vi "Write OCP_Enable.vi"(8 "error in":errorcluster, 10 "OCP_Enable":bool, 11 "36234A in":refnum<class "36234A.lvclass">) -> (0 "error out":errorcluster, 3 "36234A out":refnum<class "36234A.lvclass">)   [LabVIEW 2019, in "36234A.lvlib" / "36234A.lvclass"]
uses:
  Library/36234A.lvclass
  C:/Users/Public/Documents/Development/builds/Instruments/PowerSupply.lvlibp/Library/PowerSupply.lvclass
  Library/36234A.lvclass/36234A.ctl
  builds/Instruments/PowerSupply.lvlibp/Accessors/Read Active Channel.vi
  builds/Instruments/PowerSupply.lvlibp/Library/PowerSupply.lvclass
  <instrlib>/Keysight E36000 Series/Keysight E36000 Series.lvlib
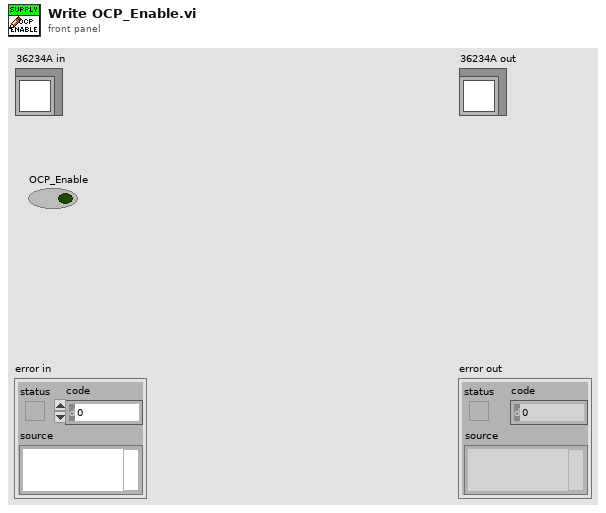
[diagram p1: front panel]
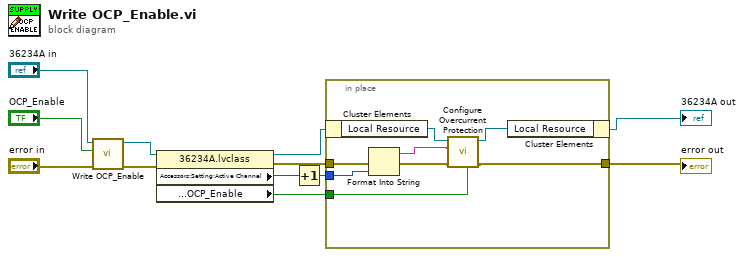
[diagram p0: block diagram]
diagram:
  n1 = call-parent "Write OCP_Enable.vi"("error in"="error in", "OCP_Enable"="OCP_Enable", "PowerSupply in"="36234A in") -> ("error out"=w4:errorcluster, "PowerSupply out"=w3:refnum<class "36234A.lvclass">)  [unwired: 7 in]
  n2 = property class="36234A.lvclass"(reference=w3, error in=w4) -> (reference out=w7:refnum<class "36234A.lvclass">, error out=w8:errorcluster, "Accessors:Setting:Active Channel"=w6:u32, "Accessors:Setting:Protection:OCP_Enable"=w9:bool)
  n3 = Increment(x=w6) -> (x+1=w5:u32)
  n4 = in-place {
    in-place-border: w8 -> [w19]
    in-place-border: [w16] -> w1
    in-place-border: w5 -> [w20]
    in-place-border: w9 -> [w13]
    n5 = in-place-cluster #1(w7) -> ("Local Resource"=w18:refnum<visa-resource-name>)
    n6 = Format Into String(error in=w19, w20) -> (resulting string=w14:string, error out=w15:errorcluster)  [unwired: 2 in]
    n7 = call <instrlib>:"Configure Overcurrent Protection.vi"("Enable Current Protection (T: Enable)"=w13, "error in (no error)"=w15, "Channel (1)"=w14, "VISA resource name"=w18) -> ("error out"=w16:errorcluster, "VISA resource name out"=w17:refnum<visa-resource-name>)  [unwired: 6 in]
    n8 = in-place-cluster #1("Local Resource"=w17) -> (→"36234A out":refnum<class "36234A.lvclass">)
  }
  "error out" <- w1
